vi "Commit Properties.vi"   [LabVIEW 2020, in "SLSC.lvlib"]
doc: "Commits all properties with pending changes to hardware, for the specified resource(s). If you set a property multiple times between commits, only the last value will be committed."
uses:
  <vilib>/SLSC/SLSC.lvlib
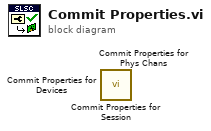
[diagram p0: block diagram]
diagram:
  n1 = call <vilib>:"Commit Properties for Session.vi"() -> ()  [unwired: 14 in, 2 out]
  n2 = call <vilib>:"Commit Properties for Phys Chans.vi"() -> ()  [unwired: 14 in, 2 out]
  n3 = call <vilib>:"Commit Properties for Devices.vi"() -> ()  [unwired: 14 in, 2 out]
